vi "Webcam.vi"(8 "error in (no error)":errorcluster, 10 "Image Name":string="webcam", 11 "Session In":T2="cam0") -> (0 "error out":errorcluster, 3 "Image":T1(plugin-control))   [LabVIEW 2014]
uses:
  <vilib>/userdefined/High Color/IMAQdx.ctl
  <vilib>/vision/driver/NI_Vision_Acquisition_Software.lvlib
panel:
  in  "Boolean":bool
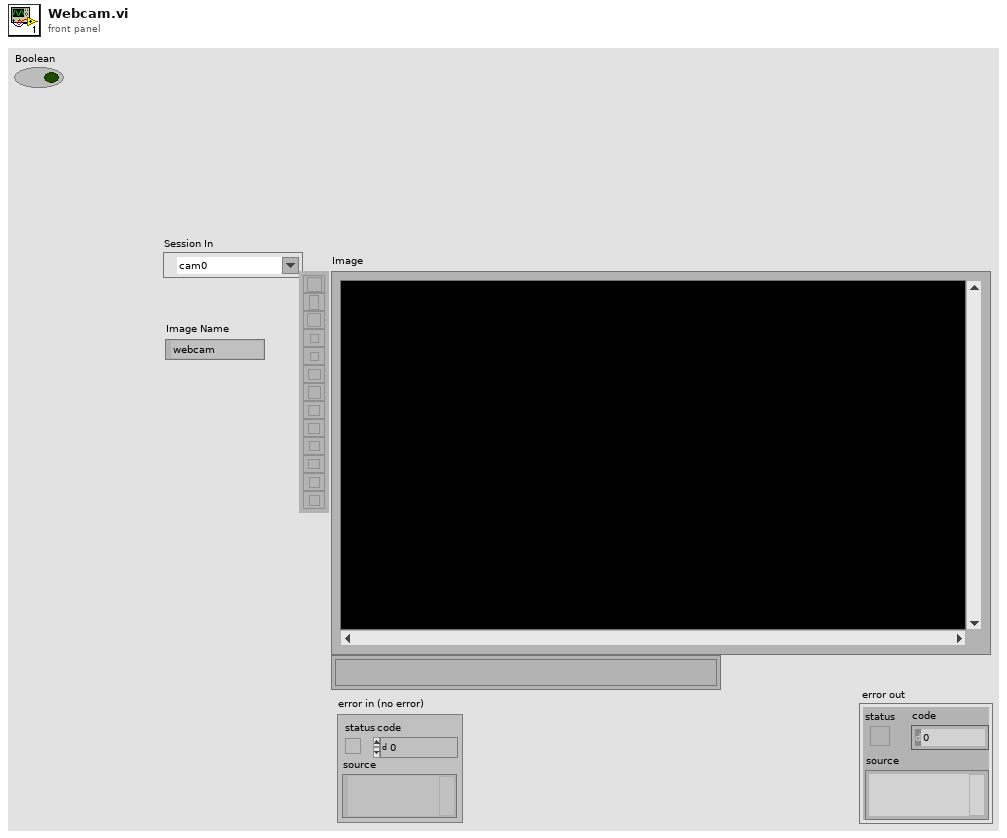
[diagram p1: front panel]
types:
  T1 = typedef "IMAQ Image.ctl" = refnum<image>
  T2 = typedef "IMAQdx.ctl" = refnum<k21>
  T3 = typedef "Image Type" = u32
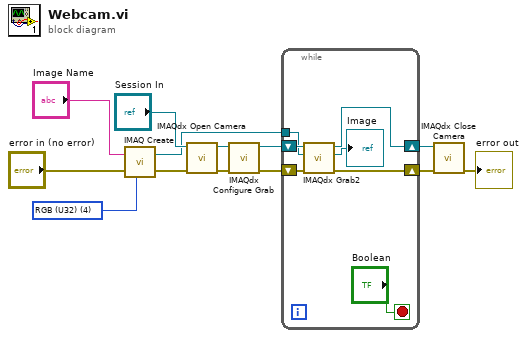
[diagram p0: block diagram]
diagram:
  w6 = T3 4 items=["Grayscale (U8)", "Grayscale (I16)", "Grayscale (SGL)", "Complex (CSG)", "RGB (U32)", "HSL (U32)", "RGB (U64)", "Grayscale (U16)"] ("Image Type")
  n1 = call "IMAQ Create"("Image Name"="Image Name", "Image Type"=w6, "error in (no error)"="error in (no error)") -> ("New Image"=w5:T1, "error out"=w3:errorcluster)  [unwired: 2 in]
  n2 = call <vilib>:"IMAQdx Open Camera.vi"("error in"=w3, "Session In"="Session In") -> ("error out"=w9:errorcluster, "Session Out"=w10:T2)  [unwired: 8 in]
  n3 = call <vilib>:"IMAQdx Configure Grab.vi"("error in"=w9, "Session In"=w10) -> ("error out"=w11:errorcluster, "Session Out"=w12:T2)  [unwired: 8 in]
  n4 = while {
    tunnel: w5 -> [w16]
    shift-right: [w17] -> w7
    shift-left: w12 -> [w19]
    shift-right: [w20] -> w13
    shift-left: w11 -> [w18]
    stop <- "Boolean" stop-if-true
    n5 = call <vilib>:"IMAQdx Grab2.vi"("error in"=w18, "Image In"=w16, "Session In"=w19) -> ("error out"=w20:errorcluster, "Image Out"=→"Image":T1, "Session Out"=w17:T2)  [unwired: 5 in, 1 out]
  }
  n6 = call <vilib>:"IMAQdx Close Camera.vi"("error in"=w13, "Session In"=w7) -> ("error out"=→"error out":errorcluster)  [unwired: 9 in]
